vi "interfaz-grafica - Final.vi"() -> ()   [LabVIEW 2024]
uses:
  VI - Juan Diego/160620 Optotune Lens Driver 4 Labview package/Hello Optotune Lens (30.06.2015)/Calibration.ctl
  <vilib>/vision/Avi.llb/IMAQ AVI2 Refnum.ctl
  <vilib>/Instr/_visa.llb/VISA Configure Serial Port (Instr).vi
  <vilib>/Utility/file.llb/Write Delimited Spreadsheet (string).vi
  <vilib>/Utility/file.llb/Read Delimited Spreadsheet (string).vi
  <vilib>/Utility/inputDevices.llb/mouseAcquire.vi
  <vilib>/Utility/inputDevices.llb/closeMouse.vi
  <vilib>/vision/NI_Vision_Development_Module.lvlib
panel:
  in  "RECIVE EMG SIGNAL":bool
  in  "Server Closed":string="The server VI closed the connection."
  in  "Stop":bool
  out "Waveform Graph":dbl[](graph)
  out "*(type *) &x":dbl[](array[numeric])
  out "PI_I":dbl(slide) scale=-3.0..3.0
  out "PI_D":dbl(slide) scale=-3.0..3.0
  in  "stop 7":bool
  in  "CONTROL":bool
  out "axis info":T1
  in  "stop 6":bool
  out "Vertical":i32
  out "Dioptrias Finales":dbl
  out "AVI Refnum":T2
  in  "stop 5":bool
  out "Boolean":bool
  out "Usuario 3":string(combo)
  out "Usuario 2":string(combo)
  out "USUARIO 2":string caption="USUARIO"
  out "Path Video":path
  out "Path Potencia Optica D":path
  out "Path Potencia Optica I":path
  in  "stop":bool
  out "Array 2":dbl[](array[numeric])
  out "Array":dbl[](array[numeric])
  out "Path DATOS":path
  in  "stop 2":bool
  out "Path":path=path "C:/Users/willi/GITHUB/TG/OBJ 2 - RECOLECCION DE DATOS/registro-usuarios.csv"
  out "error out":errorcluster
  in  "Tab Control":enum32{"Experimento", "Configuración"}(tab)
  in  "LED-IR":bool
  out "REC":bool
  in  "ADQUIRIR":bool
  in  "DETENER":bool
  out "DPT  IZQ":dbl
  out "DPT  DER":dbl
  out "Potencia  Ojo Derecho":dbl[](graph)
  out "ROI (Ojo)":T3(plugin-control)
  out "Path ADQUISICION":path
  in  "Potencia inicial lente derecho":dbl(slide) scale=-3.0..3.0
  in  "Potencia inicial lente izquierdo":dbl(slide) scale=-3.0..3.0
  out "Full Image":T3(plugin-control)
  in  "VISA resource name 3":refnum<visa-resource-name>
  in  "Tab Control 2":T4(tab)
  in  "Usuario":string(combo)
  in  "registrarButtom":bool
  in  "Cluster":T5 {"Fecha de nacimiento" format="%<%x>T"}
  out "Nuevo Usuario":i32
  out "USUARIO":string
  in  "VISA resource name 4":refnum<visa-resource-name>
  in  "VISA Arduino":refnum<visa-resource-name>
  out "error out 4":errorcluster
  out "error out 3":errorcluster
  in  "stop 4":bool
  in  "error in (no error) 3":errorcluster
  in  "error in (no error) 4":errorcluster
  in  "stop 3":bool
  out "VISA resource name out 2":string
  out "Command to Port":string
  out "Data":string
  out "OK":bool
  out "Calibration 2":T6 {"Max Current A" format="%#_g mA"; "Max Current B" format="%#_g mA"; "UCL A" format="%#_g mA"; "LCL A" format="%#_g mA"; "UCL B" format="%#_g mA"; "LCL B" format="%#_g mA"}
  out "VISA resource name out":string
  out "ID":u16
  in  "Calibration":T6={"Max Current A"=293.0, "Max Current B"=293.0, "UCL A"=300.0, "UCL B"=300.0, "LCL A"=0.0, "LCL B"=0.0} {"Max Current A" format="%#_g mA"; "Max Current B" format="%#_g mA"; "UCL A" format="%#_g mA"; "LCL A" format="%#_g mA"; "UCL B" format="%#_g mA"; "LCL B" format="%#_g mA"}
  # "Seleccione la Region de Interes (ROI. el ojo)"
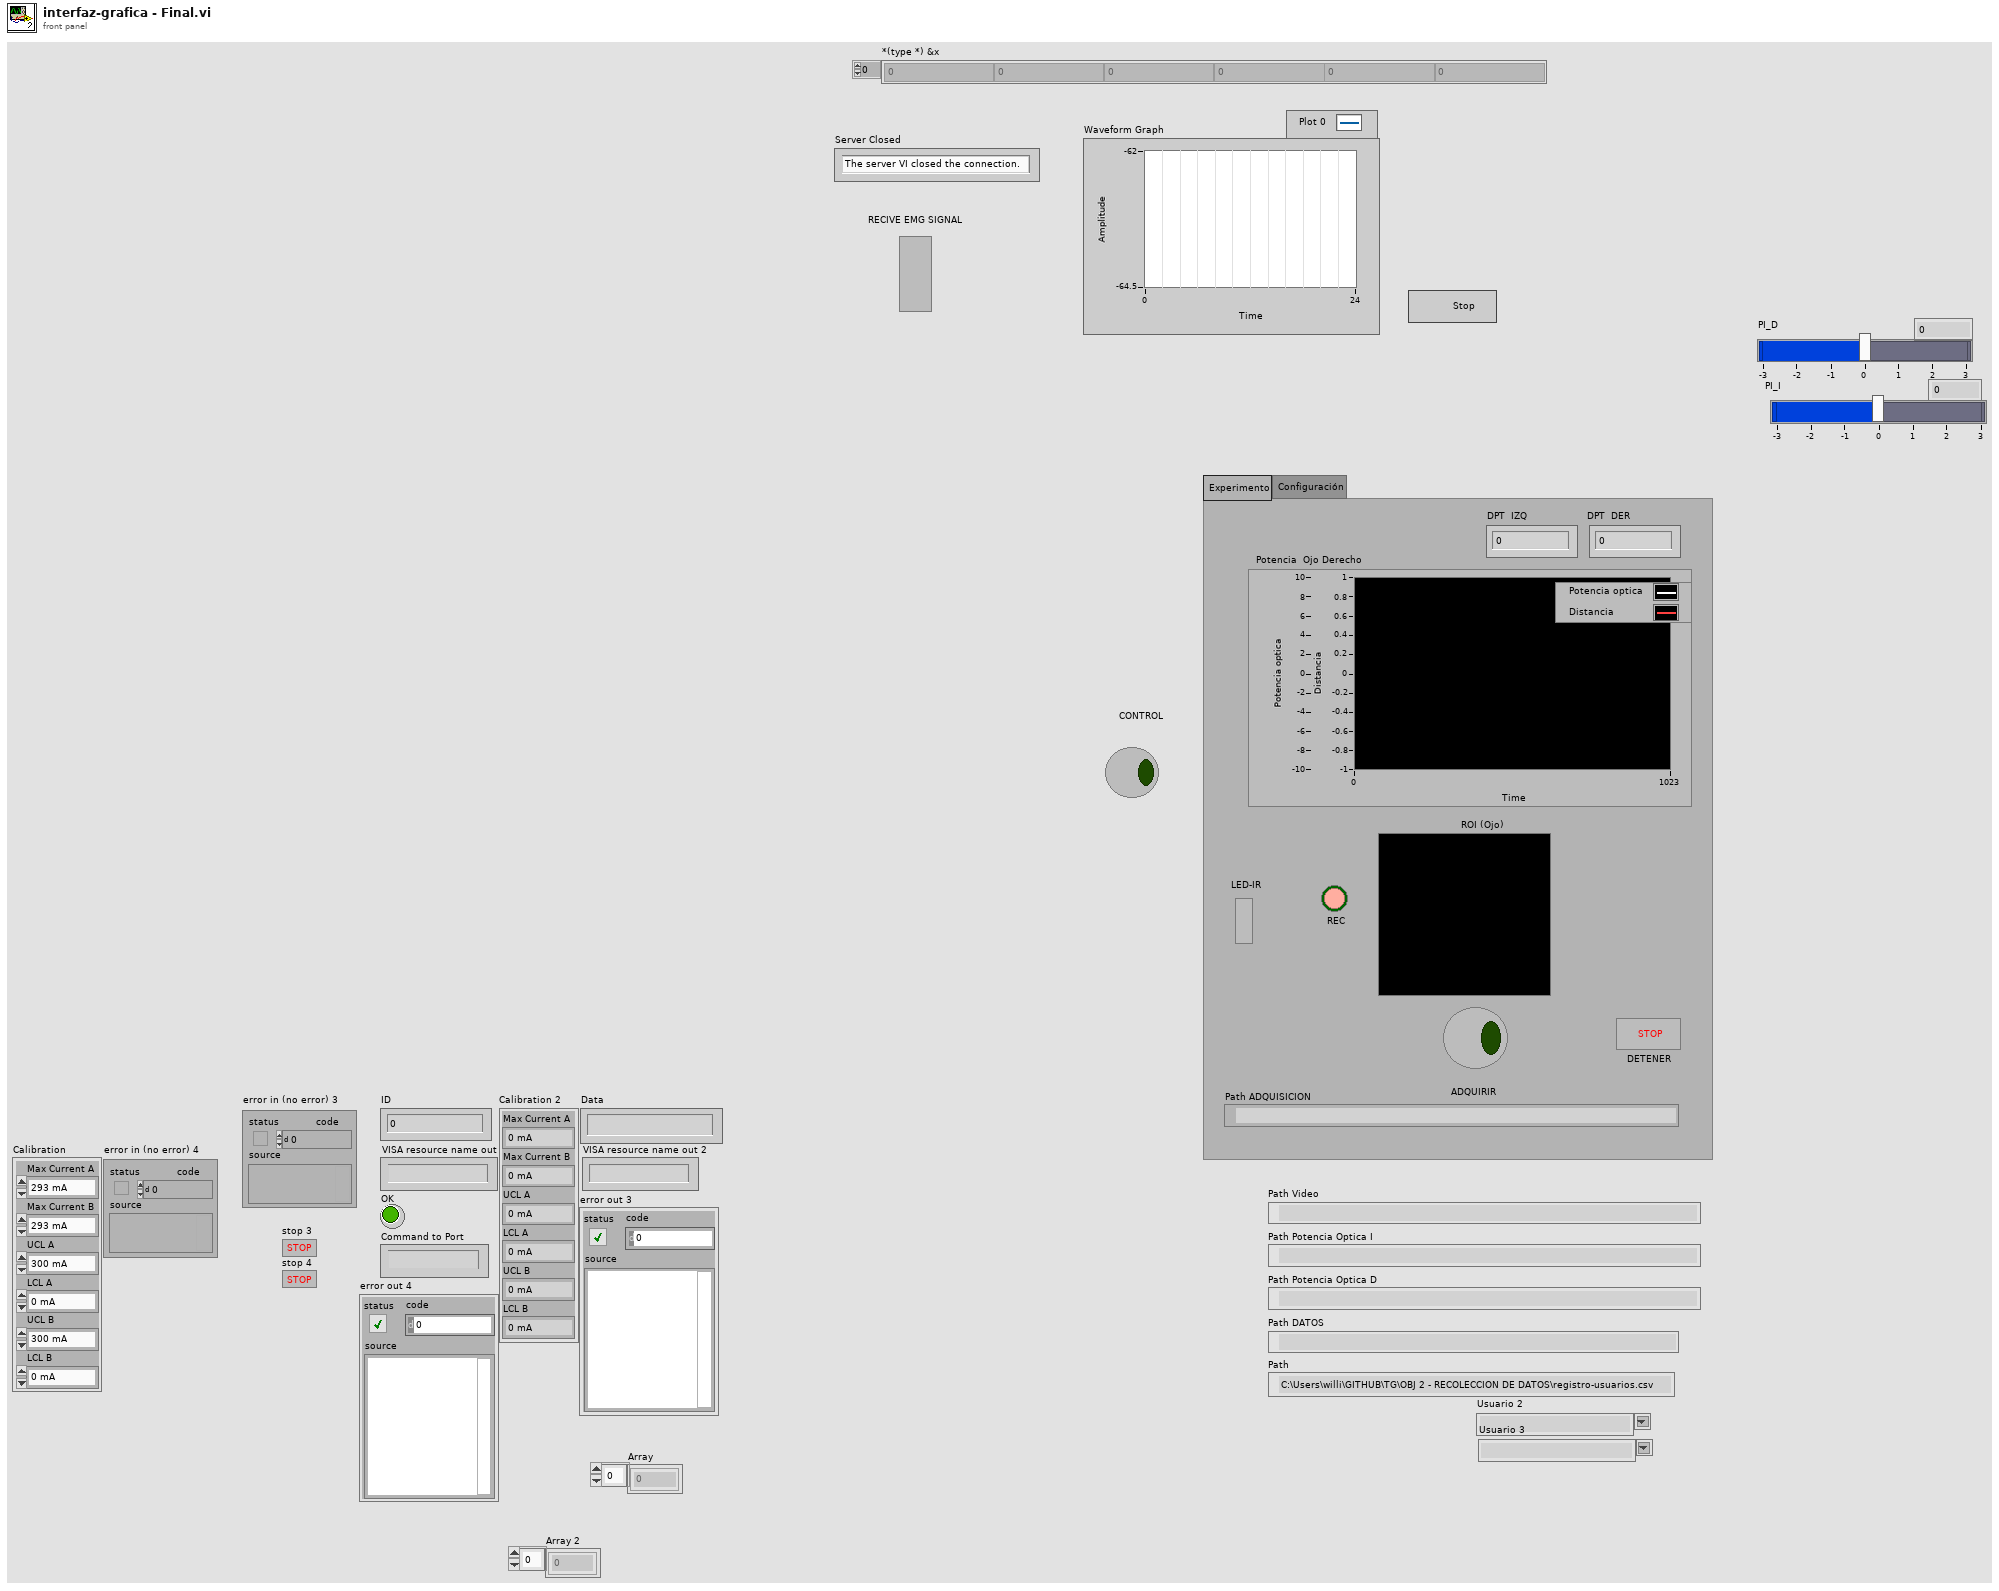
[diagram p1: front panel]
types:
  T1 = cluster{"Horizontal":i32, "Vertical":i32, "Scrolling":i32}
  T2 = typedef "IMAQ AVI2 Refnum.ctl" = refnum<k20>
  T3 = typedef "IMAQ Image.ctl" = refnum<image>
  T4 = enum32{"Seleccionar Usuario", "Registrar Nuevo Usuario"}
  T5 = cluster{"Fecha de nacimiento":timestamp, "Genero":enum16{"Mujer", "Hombre"}, "Error Refractivo":enum16{"No sabe", "Miopia", "Hipermetropia", "No tiene"}}
  T6 = typedef "Calibration.ctl" = cluster{"Max Current A":dbl, "Max Current B":dbl, "UCL A":dbl, "UCL B":dbl, "LCL A":dbl, "LCL B":dbl}
  T7 = typedef "Image Type" = u32
  T8 = cluster{"Global Rectangle":i32[], "Contours":cluster{"Contour Type":u32, "ROI Type":u32, "Points":i32[]}[]}
  T9 = cluster{"Numero \nUsuario":i32, "Fecha de nacimiento":timestamp, "Genero":enum16{"Mujer", "Hombre"}, "Error Refractivo":enum16{"No sabe", "Miopia", "Hipermetropia", "No tiene"}}
  T10 = enum16{"No sabe", "Miopia", "Hipermetropia", "No tiene"}
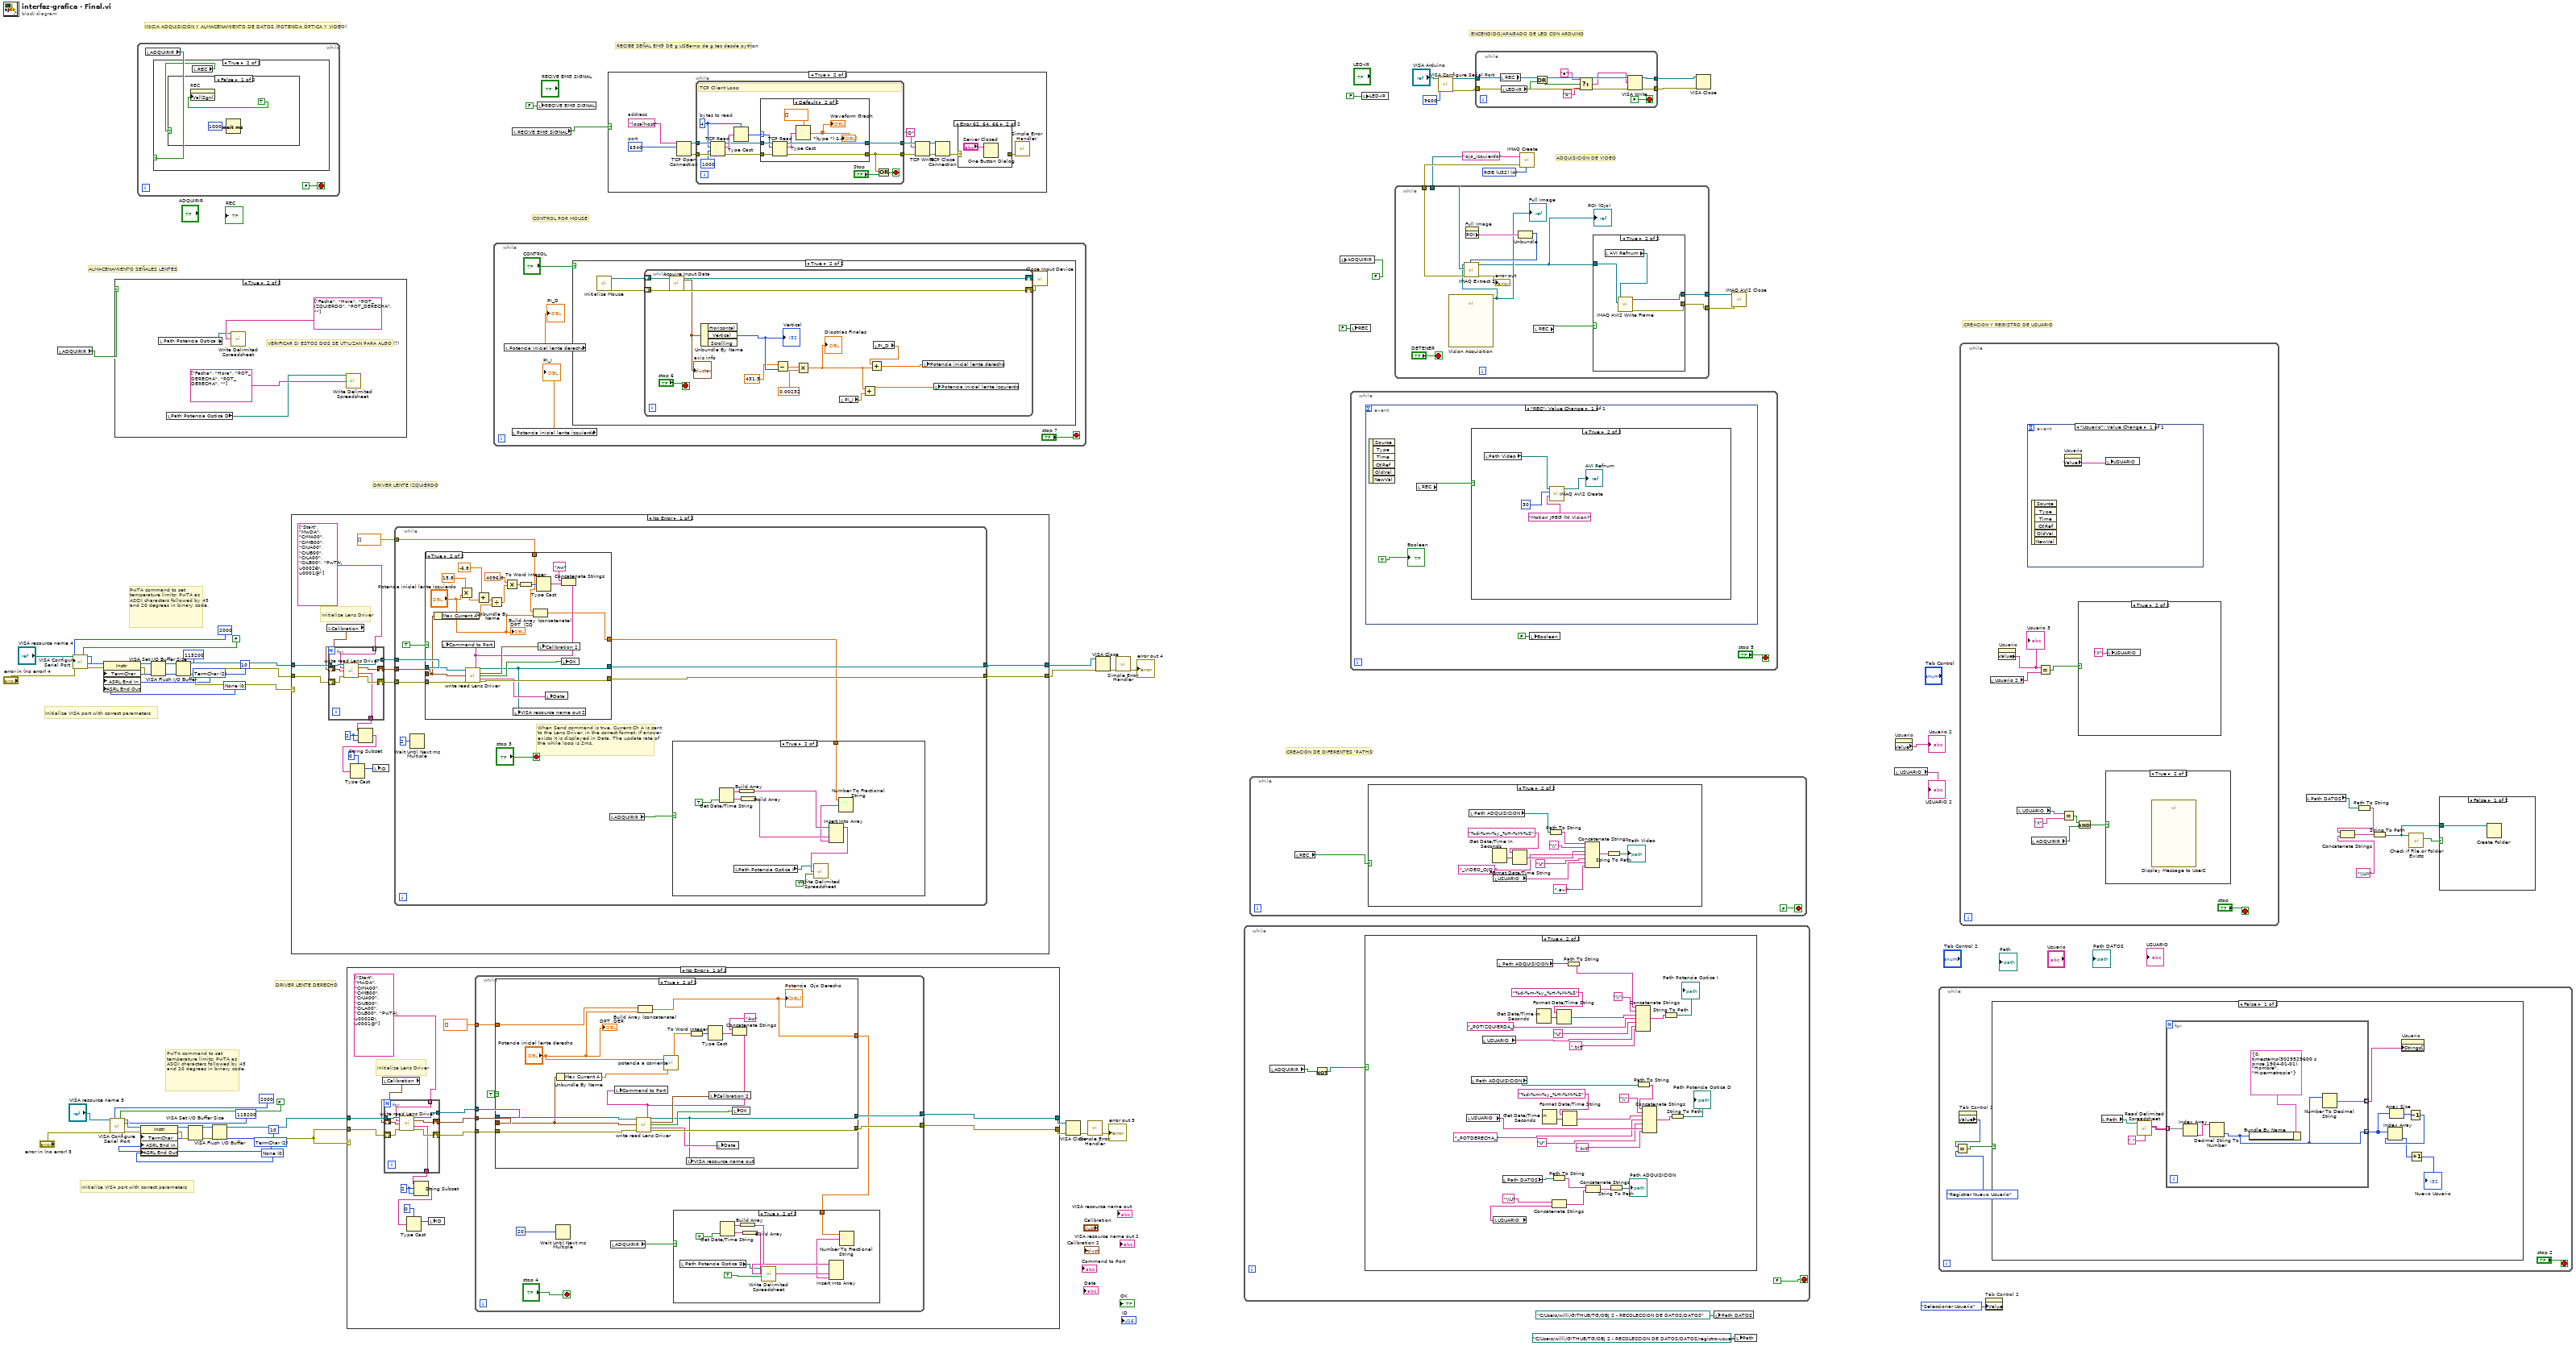
[diagram p0: block diagram]
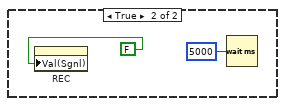
[diagram p6: hidden frame]
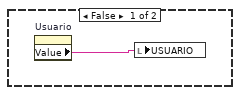
[diagram p12: hidden frame]
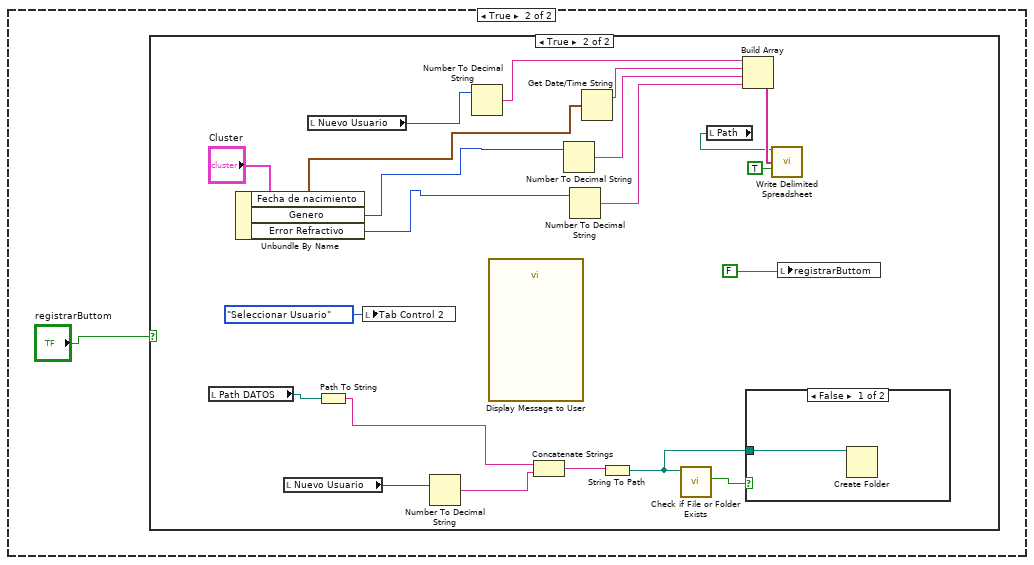
[diagram p15: hidden frame]
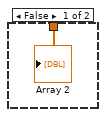
[diagram p19: hidden frame]
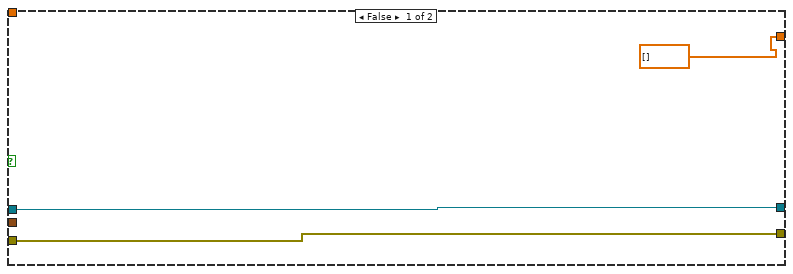
[diagram p20: hidden frame]
diagram:
  w30 = T7 4 items=["Grayscale (U8)", "Grayscale (I16)", "Grayscale (SGL)", "Complex (CSG)", "RGB (U32)", "HSL (U32)", "RGB (U64)", "Grayscale (U16)"] ("Image Type")
  w51 = u16 0 items=["None", "Last Bit", "TermChar", "Break"] ("Serial Settings:End Mode for Writes")
  w50 = u16 2 items=["None", "Last Bit", "TermChar"] ("Serial Settings:End Mode for Reads")
  w63 = u16 0 items=["None", "Last Bit", "TermChar", "Break"] ("Serial Settings:End Mode for Writes")
  w62 = u16 2 items=["None", "Last Bit", "TermChar"] ("Serial Settings:End Mode for Reads")
  # "RECIBE SEÑAL EMG DE g.USBamp de g.tec desde python"
  # "ENCENDIDO/APAGADO DE LED CON ARDUINO"
  # "INICIA ADQUISICIÓN Y ALMACENAMIENTO DE DATOS (POTENCIA ÓPTICA Y VIDEO)"
  # "ADQUISICIÓN DE VIDEO"
  # "CREACION Y REGISTRO DE USUARIO"
  # "CREACIÓN DE DIFERENTES 'PATHS'"
  # "ALMACENAMIENTO SEÑALES LENTES"
  # "DRIVER LENTE DERECHO"
  # "DRIVER LENTE IZQUIERDO"
  # "CONTROL POR MOUSE"
  # "PwTA command to set temperature limits: PwTA as ASCII characters followed by 45 and 20 degrees in binary code."
  # "Initialize VISA port with correct parameters"
  # "PwTA command to set temperature limits: PwTA as ASCII characters followed by 45 and 20 degrees in binary code."
  # "Initialize VISA port with correct parameters"
  n1 = local read "ADQUIRIR"() -> (w22:bool)
  n2 = call-poly "VISA Configure Serial Port"("VISA resource name"="VISA resource name 4", "timeout (10sec)"=u32 2000, "Enable Termination\nChar (T)"=FALSE ("Enable Termination\nChar (T)"), "baud rate (9600)"=u32 115200, "error in (no error)"="error in (no error) 4") -> ("VISA resource name out"=w58:refnum<visa-resource-name>, "error out"=w60:errorcluster)  [unwired: 9 in]
  n3 = property class="Instr"(reference=w58, error in=w60, "TermChar"=u8 10 ("Message Based Settings:Termination Character"), "ASRL End In"=w62, "ASRL End Out"=w63) -> (reference out=w59:refnum<visa-resource-name>, error out=w61:errorcluster)
  n4 = call-poly "VISA Configure Serial Port"("VISA resource name"="VISA resource name 3", "timeout (10sec)"=u32 2000, "Enable Termination\nChar (T)"=FALSE ("Enable Termination\nChar (T)"), "baud rate (9600)"=u32 115200, "error in (no error)"="error in (no error) 3") -> ("VISA resource name out"=w46:refnum<visa-resource-name>, "error out"=w48:errorcluster)  [unwired: 9 in]
  n5 = case shown="True" w22 {
    frame False {
    }
    frame True {
      # "VERIFICAR SI ESTOS DOS SE UTILIZAN PARA ALGO (?)"
      n6 = local read "Path Potencia Optica I"() -> (w71:path)
      n7 = local read "Path Potencia Optica D"() -> (w70:path)
      n8 = call-poly <vilib>:"Write Delimited Spreadsheet.vi"("file path (dialog if empty)"=w71, "1D data"=string[] ["Fecha", "Hora", "POT_IZQUIERDO", "POT_DERECHA", ""]) -> ()  [unwired: 12 in, 2 out]
      n9 = call-poly <vilib>:"Write Delimited Spreadsheet.vi"("file path (dialog if empty)"=w70, "1D data"=string[] ["Fecha", "Hora", "POT_DERECHA", "POT_DERECHA", ""]) -> ()  [unwired: 12 in, 2 out]
    }
  }
  n10 = while {
    stop <- FALSE stop-if-true
    n11 = local read "ADQUIRIR"() -> (w74:bool)
    n12 = case shown="True" w74 {
      frame False {
      }
      frame True {
        n13 = local read "REC"() -> (w76:bool)
        n14 = case shown="False" w76 {
          frame False {
            n15 = property on="REC" class="Bool (strict)"("Val(Sgnl)"=TRUE ("Value (Signaling)")) -> ()  [unwired: 2 in, 2 out]
            n16 = Wait (ms)(milliseconds to wait=u32 1000) -> ()  [unwired: 1 out]
          }
          frame True {
            n17 = property on="REC" class="Bool (strict)"("Val(Sgnl)"=FALSE ("Value (Signaling)")) -> ()  [unwired: 2 in, 2 out]
            n18 = Wait (ms)(milliseconds to wait=u32 5000) -> ()  [unwired: 1 out]
          }
        }
      }
    }
  }
  n19 = property class="Instr"(reference=w46, error in=w48, "TermChar"=u8 10 ("Message Based Settings:Termination Character"), "ASRL End In"=w50, "ASRL End Out"=w51) -> (reference out=w47:refnum<visa-resource-name>, error out=w49:errorcluster)
  n20 = VISA Set I/O Buffer Size(VISA resource name=w59, error in (no error)=w61) -> (VISA resource name out=w65:refnum<visa-resource-name>, error out=w66:errorcluster)  [unwired: 2 in]
  n21 = VISA Flush I/O Buffer(VISA resource name=w65, error in (no error)=w66) -> (VISA resource name out=w68:refnum<visa-resource-name>, error out=w67:errorcluster)  [unwired: 1 in]
  n22 = VISA Set I/O Buffer Size(VISA resource name=w47, error in (no error)=w49) -> (VISA resource name out=w53:refnum<visa-resource-name>, error out=w54:errorcluster)  [unwired: 2 in]
  n23 = VISA Flush I/O Buffer(VISA resource name=w53, error in (no error)=w54) -> (VISA resource name out=w41:refnum<visa-resource-name>, error out=w40:errorcluster)  [unwired: 1 in]
  n24 = case shown="No Error" w67 {
    tunnel: w67 -> [w95 w152]
    tunnel: w68 -> [w94 w153]
    tunnel: [w93 w152] -> w33
    tunnel: [w92 w153] -> w32
    frame No Error {
      w91 = 2 ("length (rest)")
      # "Initialize Lens Driver"
      n25 = local read "Calibration"() -> (w83:T6)
      n26 = for {
        tunnel: w94 -> [w150]
        tunnel: [w147] -> w86
        tunnel: string[] ["Start", "MwDA", "CrMA00", "CrMB00", "CrUA00", "CrUB00", "CrLA00", "CrLB00", "PwTA\u0002Ð\u0001@"] -> [w145] mode=indexing
        tunnel: [w144] -> w85
        shift-right: [w148] -> w87
        shift-left: w83 -> [w149]
        shift-right: [w146] -> w88
        shift-left: w95 -> [w151]
        n27 = call "write read Lens Driver.vi"("VISA resource name"=w150, "command"=w145, "Calibration"=w149, "error in (no error)"=w151) -> ("VISA resource name out"=w147:refnum<visa-resource-name>, "Calibration 2"=w148:T6, "Data"=w144:string, "error out"=w146:errorcluster)  [unwired: 4 in, 4 out]
      }
      n28 = String Subset(string=w85, offset (0)=w91, length (rest)=w91) -> (substring=w89:string)
      n29 = Type Cast(type=u16 0 ("length (rest)"), x=w89) -> (*(type *) &x=w84:u16)
      n30 = local write "ID"(w84) -> ()
      n31 = while {
        tunnel: [w100] -> w93
        tunnel: [w101] -> w92
        tunnel: w88 -> [w106]
        tunnel: w87 -> [w105]
        tunnel: w86 -> [w104]
        tunnel: dbl[] [] -> [w97]
        stop <- "stop 3" stop-if-true
        # "When Send command is true, Current Ch A is sent to the Lens Driver, in the correct format. If answer exists it is displayed in Data. The update rate of the while loop is 2ms."
        n32 = Wait Until Next ms Multiple(millisecond multiple=u32 2) -> ()  [unwired: 1 out]
        n33 = case shown="True" TRUE ("Send command") {
          tunnel: [w120 w143] -> w100
          tunnel: w106 -> [w120 w142]
          tunnel: w105 -> [_ w130]
          tunnel: w104 -> [w119 w141]
          tunnel: [w119 w131] -> w101
          tunnel: [dbl[] [] w121] -> w98
          tunnel: w97 -> [_ w123]
          frame False {
          }
          frame True {
            n34 = Unbundle By Name(w130) -> ("Max Current A"=w129:dbl)
            n35 = Multiply(x=15.8, y="Potencia inicial lente izquierdo") -> (x*y=w127:dbl)
            n36 = Add(x=-6.8, y=w127) -> (x+y=w125:dbl)
            n37 = Divide(x=w125, y=w129) -> (x/y=w128:dbl)
            n38 = Multiply(x=4096.0, y=w128) -> (x*y=w139:dbl)
            n39 = To Word Integer(number=w139) -> (16bit integer=w138:i16)
            n40 = Build Array (concatenate)(w123, "Potencia inicial lente izquierdo") -> (w121:dbl[])
            n41 = Type Cast(x=w138) -> (*(type *) &x=w137:string)  [unwired: 1 in]
            n42 = Concatenate Strings("Aw", w137) -> (w133:string)
            n43 = local write "Command to Port"(w133) -> ()
            n44 = call "write read Lens Driver.vi"("VISA resource name"=w141, "command"=w133, "Calibration"=w130, "error in (no error)"=w142) -> ("VISA resource name out"=w131:refnum<visa-resource-name>, "Calibration 2"=w135:T6, "OK"=w134:bool, "Data"=w132:string, "error out"=w143:errorcluster)  [unwired: 4 in, 3 out]
            n45 = local write "VISA resource name out 2"(w131) -> ()
            n46 = local write "Calibration 2"(w135) -> ()
            n47 = local write "Data"(w132) -> ()
            n48 = local write "OK"(w134) -> ()
            "DPT  IZQ" <- "Potencia inicial lente izquierdo"
          }
        }
        n49 = local read "ADQUIRIR"() -> (w96:bool)
        n50 = case shown="True" w96 {
          tunnel: w98 -> [w107 w109]
          frame False {
            "Array" <- w107
          }
          frame True {
            n51 = Get Date/Time String(want seconds? (F)=TRUE) -> (date string=w117:string, time string=w116:string)  [unwired: 2 in]
            n52 = local read "Path Potencia Optica I"() -> (w108:path)
            n53 = Build Array(w117) -> (w115:string[])
            n54 = Build Array(w116) -> (w114:string[])
            n55 = Number To Fractional String(number=w109) -> (F-format string=w110:string[])  [unwired: 3 in]
            n56 = Insert Into Array(array=w115, new element #1=w114, new element #2=w110) -> (w113:string[])  [unwired: 1 in]
            n57 = call-poly <vilib>:"Write Delimited Spreadsheet.vi"("file path (dialog if empty)"=w108, "1D data"=w113, "append to file? (new file:F)"=TRUE) -> ()  [unwired: 11 in, 2 out]
          }
        }
      }
    }
    frame Error {
    }
  }
  n58 = case shown="No Error" w40 {
    tunnel: w40 -> [w168 w219]
    tunnel: w41 -> [w167 w220]
    tunnel: [w166 w219] -> w36
    tunnel: [w165 w220] -> w37
    frame No Error {
      w164 = 2 ("length (rest)")
      # "Initialize Lens Driver"
      n59 = local read "Calibration"() -> (w156:T6)
      n60 = for {
        tunnel: w167 -> [w217]
        tunnel: [w214] -> w159
        tunnel: string[] ["Start", "MwDA", "CrMA00", "CrMB00", "CrUA00", "CrUB00", "CrLA00", "CrLB00", "PwTA\u0002Ð\u0001@"] -> [w212] mode=indexing
        tunnel: [w211] -> w158
        shift-right: [w215] -> w160
        shift-left: w156 -> [w216]
        shift-right: [w213] -> w161
        shift-left: w168 -> [w218]
        n61 = call "write read Lens Driver.vi"("VISA resource name"=w217, "command"=w212, "Calibration"=w216, "error in (no error)"=w218) -> ("VISA resource name out"=w214:refnum<visa-resource-name>, "Calibration 2"=w215:T6, "Data"=w211:string, "error out"=w213:errorcluster)  [unwired: 4 in, 4 out]
      }
      n62 = String Subset(string=w158, offset (0)=w164, length (rest)=w164) -> (substring=w162:string)
      n63 = Type Cast(type=u16 0 ("length (rest)"), x=w162) -> (*(type *) &x=w157:u16)
      n64 = local write "ID"(w157) -> ()
      n65 = while {
        tunnel: [w173] -> w166
        tunnel: [w174] -> w165
        tunnel: w161 -> [w179]
        tunnel: w160 -> [w178]
        tunnel: w159 -> [w177]
        tunnel: dbl[] [] -> [w171]
        stop <- "stop 4" stop-if-true
        n66 = case shown="True" TRUE ("Send command") {
          tunnel: [w193 w210] -> w173
          tunnel: w179 -> [w193 w209]
          tunnel: w178 -> [_ w200]
          tunnel: w177 -> [w192 w208]
          tunnel: [w192 w201] -> w174
          tunnel: w171 -> [_ w195]
          tunnel: [dbl[] [] w194] -> w170
          frame False {
          }
          frame True {
            n67 = Unbundle By Name(w200) -> ("Max Current A"=w199:dbl)
            n68 = Build Array (concatenate)(w195, "Potencia inicial lente derecho") -> (w194:dbl[])
            "Potencia  Ojo Derecho" <- w194
            n69 = call "potencia a corriente.vi"("Max current A"=w199, "Potencia"="Potencia inicial lente derecho") -> ("Corriente"=w198:dbl)
            n70 = To Word Integer(number=w198) -> (16bit integer=w207:i16)
            n71 = Type Cast(x=w207) -> (*(type *) &x=w206:string)  [unwired: 1 in]
            n72 = Concatenate Strings("Aw", w206) -> (w203:string)
            n73 = local write "Command to Port"(w203) -> ()
            n74 = call "write read Lens Driver.vi"("VISA resource name"=w208, "command"=w203, "Calibration"=w200, "error in (no error)"=w209) -> ("VISA resource name out"=w201:refnum<visa-resource-name>, "Calibration 2"=w205:T6, "OK"=w204:bool, "Data"=w202:string, "error out"=w210:errorcluster)  [unwired: 4 in, 3 out]
            n75 = local write "VISA resource name out"(w201) -> ()
            n76 = local write "Calibration 2"(w205) -> ()
            n77 = local write "Data"(w202) -> ()
            n78 = local write "OK"(w204) -> ()
            "DPT  DER" <- "Potencia inicial lente derecho"
          }
        }
        n79 = Wait Until Next ms Multiple(millisecond multiple=u32 20) -> ()  [unwired: 1 out]
        n80 = local read "ADQUIRIR"() -> (w169:bool)
        n81 = case shown="True" w169 {
          tunnel: w170 -> [w180 w182]
          frame False {
            "Array 2" <- w180
          }
          frame True {
            n82 = local read "Path Potencia Optica D"() -> (w181:path)
            n83 = Get Date/Time String(want seconds? (F)=TRUE) -> (date string=w190:string, time string=w189:string)  [unwired: 2 in]
            n84 = Build Array(w190) -> (w188:string[])
            n85 = Build Array(w189) -> (w187:string[])
            n86 = Number To Fractional String(number=w182) -> (F-format string=w183:string[])  [unwired: 3 in]
            n87 = Insert Into Array(array=w188, new element #1=w187, new element #2=w183) -> (w186:string[])  [unwired: 1 in]
            n88 = call-poly <vilib>:"Write Delimited Spreadsheet.vi"("file path (dialog if empty)"=w181, "1D data"=w186, "append to file? (new file:F)"=TRUE) -> ()  [unwired: 11 in, 2 out]
          }
        }
      }
    }
    frame Error {
    }
  }
  n89 = while {
    stop <- "stop 7" stop-if-true
    n90 = local read "Potencia inicial lente derecho"() -> (→"PI_D":dbl)
    n91 = local read "Potencia inicial lente izquierdo"() -> (→"PI_I":dbl)
    n92 = case shown="True" "CONTROL" {
      frame False {
      }
      frame True {
        n93 = call <vilib>:"Initialize Mouse.vi"() -> ("error out"=w226:errorcluster, "device ID"=w228:refnum<k1>)  [unwired: 10 in]
        n94 = while {
          shift-right: [w242] -> w227
          shift-left: w228 -> [w243]
          shift-right: [w240] -> w225
          shift-left: w226 -> [w241]
          stop <- "stop 6" stop-if-true
          n95 = call-poly <vilib>:"Acquire Input Data.vi"("device ID"=w243, "error in (no error)"=w241) -> ("device ID"=w242:refnum<k1>, "axis info"=w238:T1, "error out"=w240:errorcluster)  [unwired: 14 in, 1 out]
          "axis info" <- w238
          n96 = Unbundle By Name(w238) -> ("Vertical"=w237:i32)  [unwired: 2 out]
          "Vertical" <- w237
          n97 = Subtract(x=431.5, y=w237) -> (x-y=w235:dbl)
          n98 = Multiply(x=w235, y=0.00232) -> (x*y=w231:dbl)
          "Dioptrias Finales" <- w231
          n99 = local read "PI_I"() -> (w233:dbl)
          n100 = Add(x=w231, y=w233) -> (x+y=w229:dbl)
          n101 = local read "PI_D"() -> (w232:dbl)
          n102 = Add(x=w232, y=w231) -> (x+y=w230:dbl)
          n103 = local write "Potencia inicial lente derecho"(w230) -> ()
          n104 = local write "Potencia inicial lente izquierdo"(w229) -> ()
        }
        n105 = call-poly <vilib>:"Close Input Device.vi"("error in (no error)"=w225, "device ID"=w227) -> ()  [unwired: 8 in, 1 out]
      }
    }
  }
  n106 = local read "RECIVE EMG SIGNAL"() -> (w2:bool)
  n107 = local write "RECIVE EMG SIGNAL"(FALSE ("RECIVE EMG SIGNAL")) -> ()
  n108 = case shown="True" w2 {
    frame False {
    }
    frame True {
      w244 = u16 6340  # port
      w245 = "localhost"  # address
      n109 = TCP Open Connection(address=w245, remote port or service name=w244) -> (connection ID=w254:refnum<k5>, error out=w253:errorcluster)  [unwired: 3 in]
      n110 = while {
        tunnel: w253 -> [w264]
        tunnel: w254 -> [w265]
        tunnel: [w260] -> w251
        tunnel: [w259] -> w249
        stop <- w261 stop-if-true
        w263 = 4  # bytes to read
        # "TCP Client Loop"
        n111 = TCP Read(connection ID=w265, bytes to read=w263, error in (no error)=w264, 9:1000 ("timeout ms (25000)")) -> (connection ID out=w267:refnum<k5>, data out=w268:string, error out=w266:errorcluster)  [unwired: 1 in]
        n112 = Type Cast(type=w263, x=w268) -> (*(type *) &x=w258:i32)
        n113 = case shown="Default" w258 {
          selector: w258 -> [_ w271]
          tunnel: w267 -> [w270 w278]
          tunnel: w266 -> [w269 w277]
          tunnel: [w270 w274] -> w260
          tunnel: [w269 w273] -> w259
          frame ..0 {
            # "The server has not written any data"
          }
          frame Default {
            n114 = TCP Read(connection ID=w278, bytes to read=w271, error in (no error)=w277) -> (connection ID out=w274:refnum<k5>, data out=w272:string, error out=w273:errorcluster)  [unwired: 2 in]
            n115 = Type Cast(type=dbl[] [] ("chart"), x=w272) -> (*(type *) &x=→"Waveform Graph" →"*(type *) &x":dbl[])
          }
        }
        n116 = Or(x=w259, y="Stop") -> (x .or. y?=w261:bool)
      }
      n117 = TCP Write(connection ID=w251, data in="Q", error in (no error)=w249) -> (connection ID out=w252:refnum<k5>, error out=w250:errorcluster)  [unwired: 2 out]
      n118 = TCP Close Connection(connection ID=w252, error in (no error)=w250) -> (error out=w247:errorcluster)  [unwired: 1 in, 1 out]
      n119 = case shown="Error 62, 64, 66" w247 {
        selector: w247 -> [w255 _]
        tunnel: [w255 _] -> w246
        frame #0 {
        }
        frame #1 {
          n120 = One Button Dialog(message="Server Closed") -> ()  [unwired: 1 in, 1 out]
        }
      }
      n121 = call <vilib>:"Simple Error Handler.vi"("error in (no error)"=w246) -> ()  [unwired: 4 in, 5 out]
    }
  }
  n122 = VISA Close(VISA resource name=w37, error in (no error)=w36) -> (error out=w39:errorcluster)
  n123 = call <vilib>:"Simple Error Handler.vi"("error in (no error)"=w39) -> ("error out"=→"error out 3":errorcluster)  [unwired: 4 in, 4 out]
  n124 = VISA Close(VISA resource name=w32, error in (no error)=w33) -> (error out=w35:errorcluster)
  n125 = call <vilib>:"Simple Error Handler.vi"("error in (no error)"=w35) -> ("error out"=→"error out 4":errorcluster)  [unwired: 4 in, 4 out]
  n126 = while {
    stop <- FALSE ("stop 5") stop-if-true
    n127 = local read "ADQUIRIR"() -> (w280:bool)
    n128 = Not(x=w280) -> (.not. x?=w279:bool)
    n129 = case shown="True" w279 {
      frame False {
      }
      frame True {
        n130 = local read "USUARIO"() -> (w312:string)
        n131 = local read "Path ADQUISICION"() -> (w309:path)
        n132 = local read "USUARIO"() -> (w311:string)
        n133 = local read "USUARIO"() -> (w293:string)
        n134 = local read "Path ADQUISICION"() -> (w310:path)
        n135 = local read "Path DATOS"() -> (w294:path)
        n136 = Get Date/Time In Seconds() -> (seconds since 1Jan1904=w299:timestamp)
        n137 = Get Date/Time In Seconds() -> (seconds since 1Jan1904=w302:timestamp)
        n138 = Path To String(path=w294) -> (string=w295:string)
        n139 = Concatenate Strings("\\U" ("string"), w293) -> (w296:string)
        n140 = Format Date/Time String(time format string (%c)="%d-%m-%y_%H-%M-%S", seconds (now)=w299) -> (date/time string=w301:string)  [unwired: 1 in]
        n141 = Format Date/Time String(time format string (%c)="%d-%m-%y_%H-%M-%S", seconds (now)=w302) -> (date/time string=w304:string)  [unwired: 1 in]
        n142 = Path To String(path=w310) -> (string=w305:string)
        n143 = Concatenate Strings(w295, w296) -> (w297:string)
        n144 = String To Path(string=w297) -> (path=→"Path ADQUISICION":path)
        n145 = Concatenate Strings(w305, "\\" ("string"), w301, "_POTIZQUIERDA_" ("string"), "U" ("string"), w311, ".txt" ("string")) -> (w300:string)
        n146 = Path To String(path=w309) -> (string=w306:string)
        n147 = Concatenate Strings(w306, "\\" ("string"), w304, "_POTDERECHA_" ("string"), "U" ("string"), w312, ".txt" ("string")) -> (w303:string)
        n148 = String To Path(string=w300) -> (path=→"Path Potencia Optica I":path)
        n149 = String To Path(string=w303) -> (path=→"Path Potencia Optica D":path)
      }
    }
  }
  n150 = while {
    stop <- FALSE stop-if-true
    n151 = local read "REC"() -> (w313:bool)
    n152 = case shown="True" w313 {
      frame False {
      }
      frame True {
        n153 = local read "Path ADQUISICION"() -> (w320:path)
        n154 = Get Date/Time In Seconds() -> (seconds since 1Jan1904=w325:timestamp)
        n155 = local read "USUARIO"() -> (w323:string)
        n156 = Format Date/Time String(time format string (%c)="%d-%m-%y_%H-%M-%S", seconds (now)=w325) -> (date/time string=w324:string)  [unwired: 1 in]
        n157 = Path To String(path=w320) -> (string=w326:string)
        n158 = Concatenate Strings(w326, "\\" ("string"), w324, "_VIDEO_OJO_" ("string"), "U" ("string"), w323, ".avi" ("string")) -> (w322:string)
        n159 = String To Path(string=w322) -> (path=→"Path Video":path)
      }
    }
  }
  n160 = local write "ADQUIRIR"(FALSE ("ADQUIRIR")) -> ()
  n161 = while {
    stop <- "stop 5" stop-if-true
    n162 = event shown="[0] \"REC\": Value Change" {
      selector: _ -> [_]
      dyn-events: _ -> [_]
      timeout: _ -> [_]
      event "REC": Value Change {
        n163 = event-data() -> ()  [unwired: 1 in, 6 out]
        n164 = local read "REC"() -> (w329:bool)
        n165 = case shown="True" w329 {
          frame False {
          }
          frame True {
            n166 = local read "Path Video"() -> (w333:path)
            n167 = call "IMAQ AVI2 Create"("Codec"="Motion JPEG (NI Vision)", "Frames Per Second"=u32 30, "AVI Path"=w333) -> ("AVI Refnum"=→"AVI Refnum":T2)  [unwired: 7 in, 1 out]
          }
        }
        "Boolean" <- TRUE
      }
    }
    n168 = local write "Boolean"(FALSE ("Boolean")) -> ()
  }
  n169 = local write "REC"(FALSE ("REC")) -> ()
  n170 = local write "LED-IR"(FALSE ("LED-IR")) -> ()
  n171 = call-poly "VISA Configure Serial Port"("VISA resource name"="VISA Arduino", "baud rate (9600)"=u32 9600) -> ("VISA resource name out"=w7:refnum<visa-resource-name>, "error out"=w4:errorcluster)  [unwired: 12 in]
  n172 = while {
    tunnel: w7 -> [w345]
    tunnel: [w344] -> w6
    tunnel: [w343] -> w5
    tunnel: w4 -> [w342]
    stop <- FALSE stop-if-true
    n173 = local read "REC"() -> (w336:bool)
    n174 = local read "LED-IR"() -> (w335:bool)
    n175 = Or(x=w336, y=w335) -> (x .or. y?=w337:bool)
    n176 = Select(t="a", s=w337, f="b") -> (s? t:f=w339:string)
    n177 = VISA Write(VISA resource name=w345, write buffer=w339, error in (no error)=w342) -> (VISA resource name out=w344:refnum<visa-resource-name>, error out=w343:errorcluster)  [unwired: 1 out]
  }
  n178 = call "IMAQ Create"("Image Name"="ojo_izquierdo", "Image Type"=w30) -> ("New Image"=w28:T3, "error out"=w29:errorcluster)  [unwired: 3 in]
  n179 = while {
    tunnel: w29 -> [w355]
    tunnel: w28 -> [w354]
    tunnel: [w348] -> w27
    tunnel: [w347] -> w26
    stop <- "DETENER" stop-if-true
    n180 = call "Vision Acquisition"() -> ("Image Out"=w350:T3)  [unwired: 25 in, 2 out]
    "Full Image" <- w350
    n181 = property on="Full Image" class="ImageControl"() -> ("ROI"=w353:T8)  [unwired: 2 in, 2 out]
    n182 = Unbundle "Unbundle"(w353) -> ("Global Rectangle"=w352:i32[])  [unwired: 1 out]
    n183 = call "IMAQ Extract 2"("Optional Rectangle"=w352, "error in (no error)"=w355, "Image Dst"=w354, "Image Src"=w350) -> ("error out"=→"error out":errorcluster, "Image Dst Out"=w349:T3)  [unwired: 6 in]
    "ROI (Ojo)" <- w349
    n184 = local read "REC"() -> (w346:bool)
    n185 = case shown="True" w346 {
      tunnel: [_ w360] -> w348
      tunnel: [_ w359] -> w347
      tunnel: w349 -> [_ w358]
      frame False {
      }
      frame True {
        n186 = local read "AVI Refnum"() -> (w357:T2)
        n187 = call "IMAQ AVI2 Write Frame"("Image"=w358, "AVI Refnum"=w357) -> ("error out"=w360:errorcluster, "AVI Refnum (duplicate)"=w359:T2)  [unwired: 7 in, 1 out]
      }
    }
  }
  n188 = VISA Close(VISA resource name=w6, error in (no error)=w5) -> ()  [unwired: 1 out]
  n189 = local write "Path DATOS"(path "C:/Users/willi/GITHUB/TG/OBJ 2 - RECOLECCION DE DATOS/DATOS" ("Path DATOS")) -> ()
  n190 = call "IMAQ AVI2 Close"("error in (no error)"=w27, "AVI Refnum"=w26) -> ()  [unwired: 9 in, 1 out]
  n191 = local write "Path"(path "C:/Users/willi/GITHUB/TG/OBJ 2 - RECOLECCION DE DATOS/DATOS/registro-usuarios.csv" ("Path")) -> ()
  n192 = local read "USUARIO"() -> (→"USUARIO 2":string)
  n193 = property on="Usuario" class="CmbBox"() -> ("Value"=→"Usuario 2":string)  [unwired: 2 in, 2 out]
  n194 = while {
    stop <- "stop 2" stop-if-true
    n195 = property on="Tab Control 2" class="TabCtl (strict)"() -> ("Value"=w363:T4)  [unwired: 2 in, 2 out]
    n196 = Equal?(x=w363, y=T4."Registrar Nuevo Usuario") -> (x = y?=w364:bool)
    n197 = case shown="False" w364 {
      frame False {
        n198 = local read "Path"() -> (w372:path)
        n199 = call-poly <vilib>:"Read Delimited Spreadsheet.vi"("file path (dialog if empty)"=w372, "delimiter (\\t)"="," ("delimiter (\\t)")) -> ("all rows"=w371:string[][])  [unwired: 8 in, 5 out]
        n200 = for {
          tunnel: w371 -> [w378] mode=indexing
          tunnel: [w375] -> w370 mode=indexing
          tunnel: [w374] -> w365 mode=indexing
          n201 = Index Array(array=w378) -> (element=w376:string)  [unwired: 1 in]
          n202 = Decimal String To Number(string=w376) -> (number=w375:i32)  [unwired: 2 in, 1 out]
          n203 = Bundle By Name(cluster=T9 {"Numero \nUsuario"=0, "Fecha de nacimiento"=timestamp(3029529600 s since 1904-01-01), "Genero"=enum."Hombre", "Error Refractivo"=enum."Hipermetropia"} ("Cluster"), "Numero \nUsuario"=w375) -> ()  [unwired: 1 out]
          n204 = Number To Decimal String(number=w375) -> (decimal integer string=w374:string)  [unwired: 1 in]
        }
        n205 = Array Size(array=w370) -> (size(s)=w369:i32)
        n206 = property on="Usuario" class="CmbBox"("Strings[]"=w365) -> ()  [unwired: 2 in, 2 out]
        n207 = Decrement(x=w369) -> (x-1=w368:i32)
        n208 = Index Array(array=w370, index=w368) -> (element=w367:i32)
        n209 = Increment(x=w367) -> (x+1=→"Nuevo Usuario":i32)
      }
      frame True {
        n210 = case shown="True" "registrarButtom" {
          frame False {
          }
          frame True {
            n211 = local read "Path DATOS"() -> (w381:path)
            n212 = Unbundle By Name("Cluster") -> ("Fecha de nacimiento"=w390:timestamp, "Genero"=w389:enum16{"Mujer", "Hombre"}, "Error Refractivo"=w388:T10)
            n213 = local read "Nuevo Usuario"() -> (w386:i32)
            n214 = local read "Nuevo Usuario"() -> (w387:i32)
            n215 = Path To String(path=w381) -> (string=w380:string)
            n216 = local write "Tab Control 2"(T4."Seleccionar Usuario" ("Tab Control 2")) -> ()
            n217 = Number To Decimal String(number=w386) -> (decimal integer string=w385:string)  [unwired: 1 in]
            n218 = Number To Decimal String(number=w387) -> (decimal integer string=w395:string)  [unwired: 1 in]
            n219 = call "Display Message to User"() -> ()  [unwired: 10 in, 2 out]
            n220 = Concatenate Strings(w380, w385) -> (w384:string)
            n221 = Number To Decimal String(number=w389) -> (decimal integer string=w393:string)  [unwired: 1 in]
            n222 = Number To Decimal String(number=w388) -> (decimal integer string=w392:string)  [unwired: 1 in]
            n223 = Get Date/Time String(seconds (now)=w390) -> (date string=w394:string)  [unwired: 2 in, 1 out]
            n224 = String To Path(string=w384) -> (path=w383:path)
            n225 = call <vilib>:"Check if File or Folder Exists.vi"("path"=w383) -> ("file or folder exists?"=w382:bool)  [unwired: 8 in, 2 out]
            n226 = local read "Path"() -> (w399:path)
            n227 = Build Array(w395, w394, w393, w392) -> (w400:string[])
            n228 = case shown="False" w382 {
              tunnel: w383 -> [w401 _]
              frame False {
                n229 = Create Folder(path (use dialog)=w401) -> ()  [unwired: 2 in, 3 out]
              }
              frame True {
              }
            }
            n230 = call-poly <vilib>:"Write Delimited Spreadsheet.vi"("file path (dialog if empty)"=w399, "1D data"=w400, "append to file? (new file:F)"=TRUE) -> ()  [unwired: 11 in, 2 out]
            n231 = local write "registrarButtom"(FALSE ("registrarButtom")) -> ()
          }
        }
      }
    }
  }
  n232 = while {
    stop <- "stop" stop-if-true
    n233 = local read "Usuario 2"() -> (w404:string)
    n234 = property on="Usuario" class="CmbBox"() -> ("Value"=w402:string)  [unwired: 2 in, 2 out]
    "Usuario 3" <- w402
    n235 = local read "USUARIO"() -> (w406:string)
    n236 = event shown="[0] \"Usuario\": Value Change" {
      selector: _ -> [_]
      dyn-events: _ -> [_]
      timeout: _ -> [_]
      event "Usuario": Value Change {
        n237 = event-data() -> ()  [unwired: 1 in, 6 out]
        n238 = property on="Usuario" class="CmbBox"() -> ("Value"=w411:string)  [unwired: 2 in, 2 out]
        n239 = local write "USUARIO"(w411) -> ()
      }
    }
    n240 = local read "ADQUIRIR"() -> (w408:bool)
    n241 = Equal?(x=w402, y=w404) -> (x = y?=w403:bool)
    n242 = Equal?(x=w406, y="X") -> (x = y?=w407:bool)
    n243 = And(x=w407, y=w408) -> (x .and. y?=w409:bool)
    n244 = case shown="True" w403 {
      frame False {
        n245 = property on="Usuario" class="CmbBox"() -> ("Value"=w412:string)  [unwired: 2 in, 2 out]
        n246 = local write "USUARIO"(w412) -> ()
      }
      frame True {
        n247 = local write "USUARIO"("X" ("USUARIO")) -> ()
      }
    }
    n248 = case shown="True" w409 {
      frame False {
      }
      frame True {
        n249 = call "Display Message to User2"() -> ()  [unwired: 10 in, 2 out]
      }
    }
  }
  n250 = property on="Tab Control 2" class="TabCtl (strict)"("Value"=T4."Seleccionar Usuario" ("Tab Control 2")) -> ()  [unwired: 2 in, 2 out]
  n251 = local read "Path DATOS"() -> (w14:path)
  n252 = Path To String(path=w14) -> (string=w13:string)
  n253 = Concatenate Strings(w13, "\\UX" ("string")) -> (w17:string)
  n254 = String To Path(string=w17) -> (path=w16:path)
  n255 = call <vilib>:"Check if File or Folder Exists.vi"("path"=w16) -> ("file or folder exists?"=w15:bool)  [unwired: 8 in, 2 out]
  n256 = case shown="False" w15 {
    tunnel: w16 -> [w414 _]
    frame False {
      n257 = Create Folder(path (use dialog)=w414) -> ()  [unwired: 2 in, 3 out]
    }
    frame True {
    }
  }
